vi "Measure.vi"(8 "error in":errorcluster, 11 "Plugin_Driver in":refnum<class "Plugin_Driver.lvclass">) -> (0 "error out":errorcluster, 2 "Measurement Results":T1={"Voltage (V)"=1.0} {"Voltage (V)" min=-424.2 max=424.2 step=1.0 format="%#.1f"}, 3 "Plugin_Driver out":refnum<class "Plugin_Driver.lvclass">)   [LabVIEW 2020, in "Plugin.lvlib" / "Plugin_Driver.lvclass"]
doc: "This VI is a wrapper API for Instrument Driver's Measure API."
uses:
  Plugin_Driver.lvclass
  Drivers/Instrument Driver/Typedefs/Measurement Results.ctl
  Drivers/Instrument Driver/Instrument Driver.lvclass
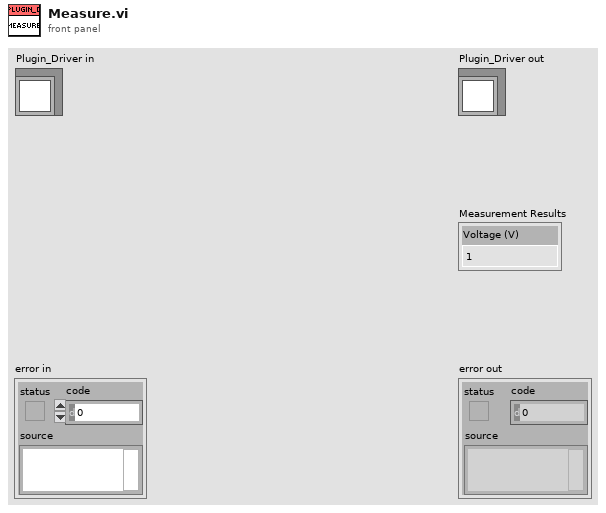
[diagram p1: front panel]
types:
  T1 = typedef "Plugin Instrument Driver.lvlib/Instrument Driver.lvclass/Measurement Results.ctl" = cluster{"Voltage (V)":dbl}
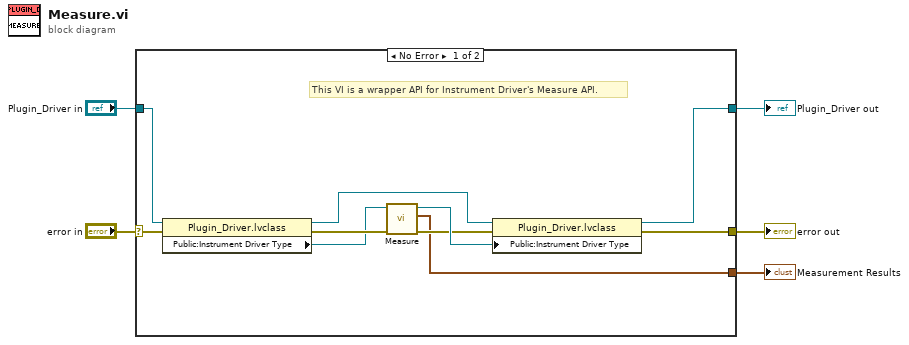
[diagram p0: block diagram]
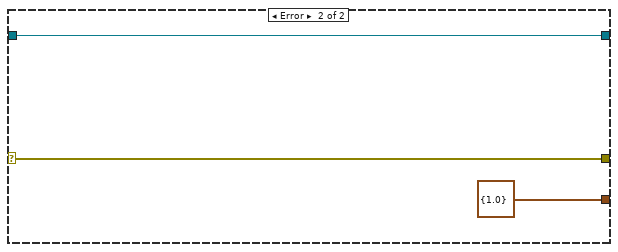
[diagram p2: hidden frame]
diagram:
  n1 = case shown="No Error" "error in" {
    selector: "error in" -> [w14 w18]
    tunnel: [w9 w18] -> w4
    tunnel: [w7 w17] -> w2
    tunnel: "Plugin_Driver in" -> [w15 w17]
    tunnel: [w6 T1 {"Voltage (V)"=1.0} ("Measurement Results")] -> w1
    frame No Error {
      # "This VI is a wrapper API for Instrument Driver's Measure API."
      n2 = property class="Plugin_Driver.lvclass"(reference=w15, error in=w14) -> (reference out=w11:refnum<class "Plugin_Driver.lvclass">, error out=w13:errorcluster, "Public:Instrument Driver Type"=w12:refnum<class "Instrument Driver.lvclass">)
      n3 = call-dynamic "Measure.vi"("error in"=w13, "Instrument Driver in"=w12) -> ("error out"=w8:errorcluster, "Measurement Results"=w6:T1, "Instrument Driver out"=w10:refnum<class "Instrument Driver.lvclass">)  [unwired: 7 in]
      n4 = property class="Plugin_Driver.lvclass"(reference=w11, error in=w8, "Public:Instrument Driver Type"=w10) -> (reference out=w7:refnum<class "Plugin_Driver.lvclass">, error out=w9:errorcluster)
    }
    frame Error {
    }
  }
  "error out" <- w4
  "Plugin_Driver out" <- w2
  "Measurement Results" <- w1
